vi "Progress Notifier.vi"(8 "error in":errorcluster) -> (0 "error out":errorcluster, 3 "notifier out":refnum<notifier>)   [LabVIEW 2013, in "LVTM.lvlib"]
uses:
  LVTM.lvlib
  Controls_LVTM/Status.ctl
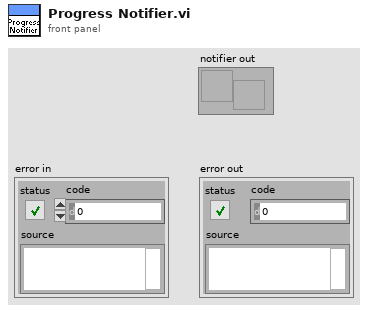
[diagram p1: front panel]
types:
  T1 = typedef "LVTM.lvlib/Status.ctl" = cluster{"Operation":string, "Total Interations":i32, "Current Iteration":i32, "Total Operations":i32, "Current Operation":i32}
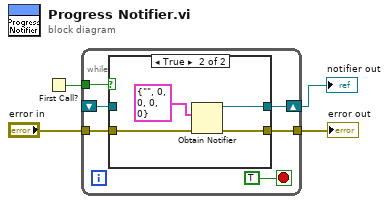
[diagram p0: block diagram]
diagram:
  n1 = First Call?() -> (First Call?: T/F=w2:bool)
  n2 = while {
    tunnel: w2 -> [w9]
    shift-right: [w8] -> w1
    shift-left: _ -> [w5]
    tunnel: "error in" -> [w7]
    tunnel: [w6] -> w4
    stop <- TRUE stop-if-true
    n3 = case shown="True" w9 {
      tunnel: [w12 w16] -> w8
      tunnel: w7 -> [w11 w15]
      tunnel: [w11 w14] -> w6
      tunnel: w5 -> [w12 _]
      frame False {
      }
      frame True {
        n4 = Obtain Notifier(notification data type=T1 {"Operation"="", "Total Interations"=0, "Current Iteration"=0, "Total Operations"=0, "Current Operation"=0}, error in (no error)=w15) -> (notifier out=w16:refnum<notifier>, error out=w14:errorcluster)  [unwired: 2 in, 1 out]
      }
    }
  }
  "error out" <- w4
  "notifier out" <- w1
